vi "AuMT8852B EDR Relative Transmit Power Extended Results.vi"(5 "Stage":T2(ring), 8 "error in (no error)":errorcluster, 11 "VISA session":refnum<visa-resource-name>) -> (0 "error out":errorcluster, 2 "error code":i32, 3 "VISA session out":refnum<visa-resource-name>, 4 "Results":T1 {"Peak 2DHx DPSK Absolute Power (dBm)" format="%.2f"; "Avg 2DHx DPSK Absolute Power (dBm)" format="%.2f"; "Min 2DHx DPSK Absolute Power (dBm)" format="%.2f"; "Max 2DHx DPSK Absolute Power (dBm)" format="%.2f"; "Peak 2DHx GFSK Absolute Power (dBm)" format="%.2f"; "Avg 2DHx GFSK Absolute Power (dBm)" format="%.2f"; "Min 2DHx GFSK Absolute Power (dBm)" format="%.2f"; "Max 2DHx GFSK Absolute Power (dBm)" format="%.2f"; "Peak 3DHx DPSK Absolute Power (dBm)" format="%.2f"; "Avg 3DHx DPSK Absolute Power (dBm)" format="%.2f"; "Min 3DHx DPSK Absolute Power (dBm)" format="%.2f"; "Max 3DHx DPSK Absolute Power (dBm)" format="%.2f"; "Peak 3DHx GFSK Absolute Power (dBm)" format="%.2f"; "Avg 3DHx GFSK Absolute Power (dBm)" format="%.2f"; "Min 3DHx GFSK Absolute Power (dBm)" format="%.2f"; "Max 3DHx GFSK Absolute Power (dBm)" format="%.2f"; "Avg power difference (dBm)" format="%.2f"; "Min power difference (dBm)" format="%.2f"; "Max power difference (dBm)" format="%.2f"; "Avg power difference (dBm)" format="%.2f"; "Min power difference (dBm)" format="%.2f"; "Max power difference (dBm)" format="%.2f"})   [LabVIEW 2017]
doc: "Anritsu MT8852B Bluetooth Tester\n\nReturns the results of the EDR Relative Transmit Power test.\n\nINPUTS\nStage - results of the individual hopping stages of the test.\n\nOUTPUTS\nResults - measurements made during the test."
panel:
  out "byte count (0)":u32=200
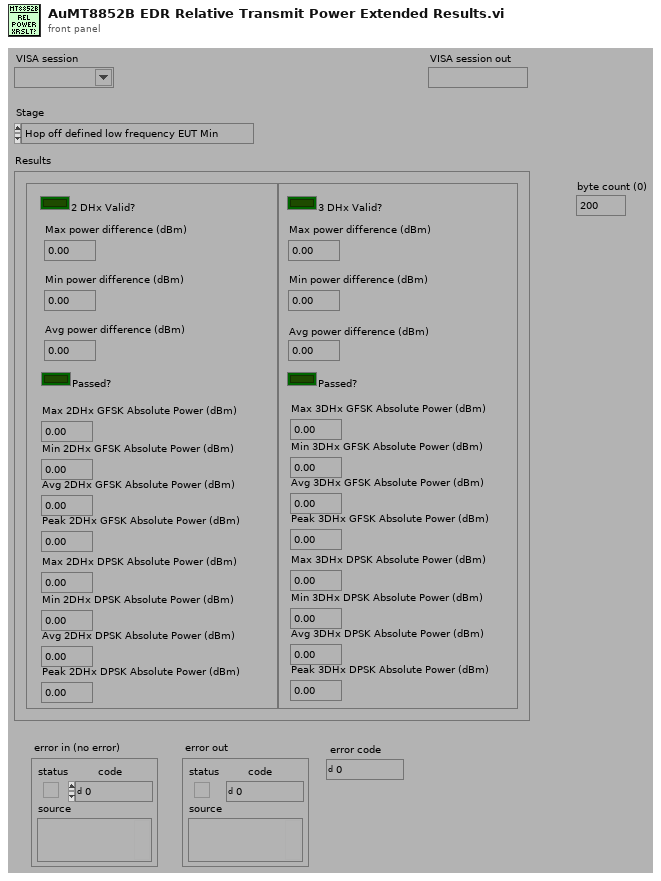
[diagram p1: front panel]
types:
  T1 = cluster{"2 DHx Valid?":bool, "Max power difference (dBm)":dbl, "Min power difference (dBm)":dbl, "Avg power difference (dBm)":dbl, "Passed?":bool, "3 DHx Valid?":bool, "Max power difference (dBm)":dbl, "Min power difference (dBm)":dbl, "Avg power difference (dBm)":dbl, "Passed?":bool, "Max 3DHx GFSK Absolute Power (dBm)":dbl, "Min 3DHx GFSK Absolute Power (dBm)":dbl, "Avg 3DHx GFSK Absolute Power (dBm)":dbl, "Peak 3DHx GFSK Absolute Power (dBm)":dbl, "Max 3DHx DPSK Absolute Power (dBm)":dbl, "Min 3DHx DPSK Absolute Power (dBm)":dbl, "Avg 3DHx DPSK Absolute Power (dBm)":dbl, "Peak 3DHx DPSK Absolute Power (dBm)":dbl, "Max 2DHx GFSK Absolute Power (dBm)":dbl, "Min 2DHx GFSK Absolute Power (dBm)":dbl, "Avg 2DHx GFSK Absolute Power (dBm)":dbl, "Peak 2DHx GFSK Absolute Power (dBm)":dbl, "Max 2DHx DPSK Absolute Power (dBm)":dbl, "Min 2DHx DPSK Absolute Power (dBm)":dbl, "Avg 2DHx DPSK Absolute Power (dBm)":dbl, "Peak 2DHx DPSK Absolute Power (dBm)":dbl}
  T2 = enum16{"Hop off defined low frequency EUT Min", "Hop off defined low frequency EUT Max", "Hop off defined medium frequency EUT Min", "Hop off defined medium frequency EUT Max", "Hop off defined high frequency EUT Min", "Hop off defined high frequency EUT Max", "Hop on defined low frequency EUT Min", "Hop on defined low frequency EUT Max", "Hop on defined medium frequency EUT Min", "Hop on defined medium frequency EUT Max", "Hop on defined high frequency EUT Min", "Hop on defined high frequency EUT Max", "Hop on all channels EUT Min", "Hop on all channels EUT Max", "Hop on any channels EUT Min", "Hop on any channels EUT Max"}
  T3 = enum16{"Simulate", "Range check", "Cache", "Query instrument status"}
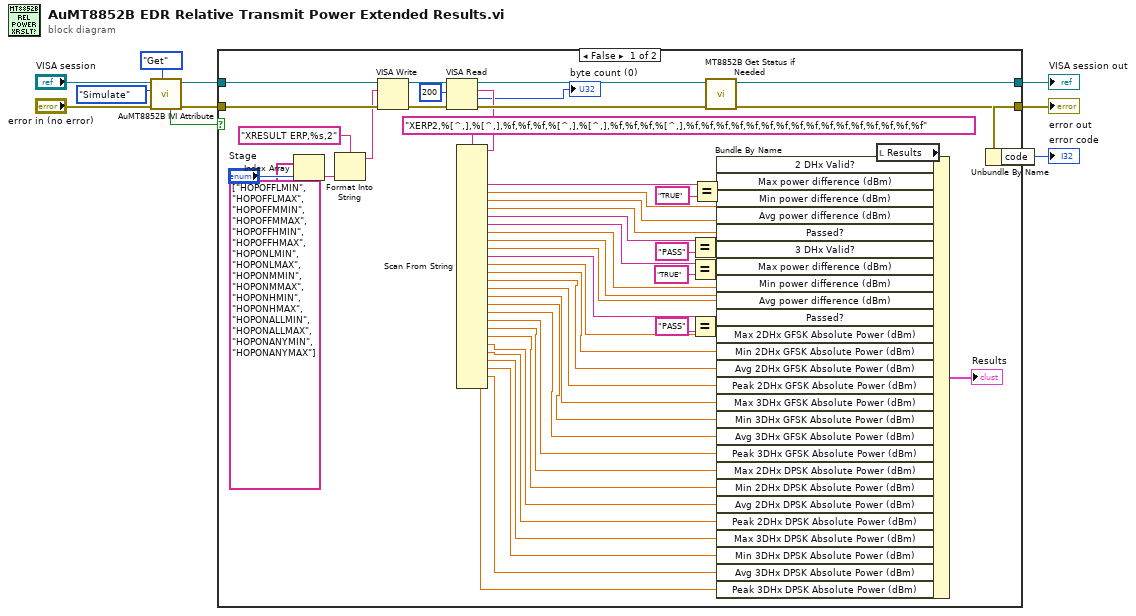
[diagram p0: block diagram]
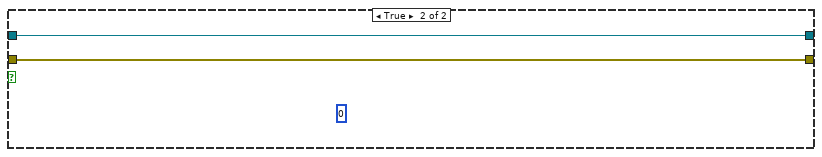
[diagram p2: hidden frame]
diagram:
  n1 = call <instrlib>:"AuMT8852B IVI Attribute.vi"("Set/Get (Set)"=enum16{"Set", "Get"}."Get", "error in (no error)"="error in (no error)", "Flag (Simulate)"=T3."Simulate", "VISA session"="VISA session") -> ("error out"=w7:errorcluster, "VISA session out"=w9:refnum<visa-resource-name>, "Value out"=w3:bool)  [unwired: 5 in]
  n2 = case shown="False" w3 {
    tunnel: [w55 w65] -> w10
    tunnel: [w54 w64] -> w1
    tunnel: w9 -> [w63 w65]
    tunnel: w7 -> [w62 w64]
    frame False {
      n3 = Index Array(array=string[] ["HOPOFFLMIN", "HOPOFFLMAX", "HOPOFFMMIN", "HOPOFFMMAX", "HOPOFFHMIN", "HOPOFFHMAX", "HOPONLMIN", "HOPONLMAX", "HOPONMMIN", "HOPONMMAX", "HOPONHMIN", "HOPONHMAX", "HOPONALLMIN", "HOPONALLMAX", "HOPONANYMIN", "HOPONANYMAX"], index="Stage") -> (element=w43:string)
      n4 = Format Into String(format string="XRESULT ERP,%s,2" ("write buffer (\"\")"), w43) -> (resulting string=w40:string)  [unwired: 2 in, 1 out]
      n5 = VISA Write(VISA resource name=w63, write buffer=w40, error in (no error)=w62) -> (VISA resource name out=w61:refnum<visa-resource-name>, error out=w60:errorcluster)  [unwired: 1 out]
      n6 = VISA Read(VISA resource name=w61, byte count=u32 200 ("byte count (0)"), error in (no error)=w60) -> (VISA resource name out=w53:refnum<visa-resource-name>, read buffer=w51:string, return count=→"byte count (0)":u32, error out=w52:errorcluster)
      n7 = Scan From String(format string="XERP2,%[^,],%[^,],%f,%f,%f,%[^,],%[^,],%f,%f,%f,%[^,],%f,%f,%f,%f,%f,%f,%f,%f,%f,%f,%f,%f,%f,%f,%f,%f" ("Format String"), input string=w51) -> (output 2=w30:string, output 3=w31:dbl, output 4=w32:dbl, output 5=w33:dbl, output 6=w38:string, output 7=w37:string, output 8=w36:dbl, output 9=w35:dbl, output 10=w34:dbl, output 11=w39:string, output 12=w29:dbl, output 13=w28:dbl, output 14=w27:dbl, output 15=w26:dbl, output 16=w25:dbl, output 17=w24:dbl, output 18=w23:dbl, output 19=w22:dbl, output 20=w21:dbl, output 21=w20:dbl, output 22=w19:dbl, output 23=w18:dbl, output 24=w17:dbl, output 25=w16:dbl, output 26=w15:dbl, output 27=w14:dbl)  [unwired: 30 in, 3 out]
      n8 = Equal?(x=w38, y="PASS") -> (x = y?=w49:bool)
      n9 = Equal?(x=w37, y="TRUE") -> (x = y?=w48:bool)
      n10 = Equal?(x=w39, y="PASS") -> (x = y?=w46:bool)
      n11 = Equal?(x=w30, y="TRUE") -> (x = y?=w50:bool)
      n12 = call <instrlib>:"MT8852B Get Status if Needed.vi"("error in (no error)"=w52, "VISA session"=w53) -> ("error out"=w54:errorcluster, "VISA session out"=w55:refnum<visa-resource-name>)  [unwired: 8 in]
      n13 = local read "Results"() -> (w13:T1)
      n14 = Bundle By Name(cluster=w13, "2 DHx Valid?"=w50, "Max power difference (dBm)"=w31, "Min power difference (dBm)"=w32, "Avg power difference (dBm)"=w33, "Passed?"=w49, "3 DHx Valid?"=w48, "Max power difference (dBm)"=w36, "Min power difference (dBm)"=w35, "Avg power difference (dBm)"=w34, "Passed?"=w46, "Max 2DHx GFSK Absolute Power (dBm)"=w29, "Min 2DHx GFSK Absolute Power (dBm)"=w28, "Avg 2DHx GFSK Absolute Power (dBm)"=w27, "Peak 2DHx GFSK Absolute Power (dBm)"=w26, "Max 3DHx GFSK Absolute Power (dBm)"=w25, "Min 3DHx GFSK Absolute Power (dBm)"=w24, "Avg 3DHx GFSK Absolute Power (dBm)"=w23, "Peak 3DHx GFSK Absolute Power (dBm)"=w22, "Max 2DHx DPSK Absolute Power (dBm)"=w21, "Min 2DHx DPSK Absolute Power (dBm)"=w20, "Avg 2DHx DPSK Absolute Power (dBm)"=w19, "Peak 2DHx DPSK Absolute Power (dBm)"=w18, "Max 3DHx DPSK Absolute Power (dBm)"=w17, "Min 3DHx DPSK Absolute Power (dBm)"=w16, "Avg 3DHx DPSK Absolute Power (dBm)"=w15, "Peak 3DHx DPSK Absolute Power (dBm)"=w14) -> (→"Results":T1)
    }
    frame True {
      (unwired) u8 0
    }
  }
  "error out" <- w1
  "VISA session out" <- w10
  n15 = Unbundle By Name(w1) -> ("code"=→"error code":i32)
